vi "Load_Destinations.vi"(8 "error in (no error)":errorcluster, 11 "AB_Application in":refnum<class "AB_Application.lvclass">) -> (0 "error out":errorcluster, 3 "AB_Application out":refnum<class "AB_Application.lvclass">)   [LabVIEW 2020, in "AB_Application.lvclass"]
uses:
  <vilib>/AppBuilder/AB_Classes/Application/AB_Application.lvclass
  e:/builds/penguin/labview/branches/2020/dev/dist/vi.lib/AppBuilder/AB_Classes/TargetFile/AB_Targetfile.lvclass
  e:/builds/penguin/labview/branches/2020/dev/dist/vi.lib/AppBuilder/AB_Classes/Build/AB_Build.lvclass
  <vilib>/AppBuilder/AB_Classes/TargetFile/AB_Targetfile.lvclass
  <vilib>/AppBuilder/AB_Classes/Build/AB_Build.lvclass
  <vilib>/AppBuilder/AB_Classes/Destination/AB_Destination.lvclass
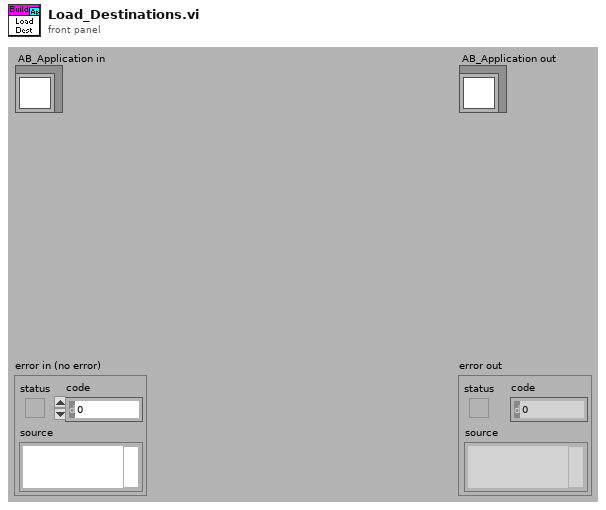
[diagram p1: front panel]
types:
  T1 = typedef "AB_Targetfile.ctl" = cluster{"targetfileName":string, "targetfileGUID":string, "enableDebugging":bool, "versionInfo":cluster{"productName":string, "legalCopyright":string, "companyName":string, "internalName":string, "fileDescription":string}, "eng_consolidatedTypeInfo":string, "fastFileFormat":bool, "eng_LEIFBuildData":u32, "versionIndependent":bool}
  T2 = typedef "AB_Build.ctl" = cluster{"buildSpecName":string, "buildSpecDescription":string, "destinations":refnum<class "AB_Destination.lvclass">[], "exclusionOption":T3, "defaultLanguage":string, "supportedLanguages":string[], "excludedDirectories":path[], "buildContext":refnum<vi>, "buildObject":T4, "preview":bool, "programatic":bool, "progressBarEvents":T5, "userLog_Path":path, "preActionID":string, "preAction_Path":path, "postActionID":string, "postAction_Path":path, "eng_checkForBrokenVIs?":bool, "eng_verboseLinkerErrors?":bool, "localDest_Path":path, "targetDest_Path":path, "removeVIObject":u16, "cache":refnum<class "PreviewCache.lvclass">, "use cache":bool, "previewCache_ID":string, "buildCache_ID":string, "eng_TempLocalDest_Path":path, "eng_collectDependencies?":bool, "versionInfo":cluster{"buildVersion":cluster{"major":u16, "minor":u16, "patch":u16, "build":u16}, "autoIncrement":bool}, "eng_enableVIChecksums":bool}
  T3 = typedef "AB_Exclusion_Option.ctl" = cluster{"typedefs":bool, "polymorphicVIs":bool, "unusedLibraryItems":bool, "modifyLibraryFile":bool, "edit-timeDependencies":bool, "inlineVIs":bool, "dependent PPLs":bool, "dependent DLLs":bool}
  T4 = typedef "ItemRef.ctl" = u64
  T5 = typedef "provcom_ProgressBar_Events.ctl" = cluster{"newJob":refnum<user-event>, "newItem":refnum<user-event>, "errorMsg":T6, "cancel":refnum<user-event>}
  T6 = typedef "mxLvBuildError.ctl" = refnum<user-event>
  T7 = typedef "AB_Destination.ctl" = cluster{"destName":string, "path":path, "libraryName":string, "preserveHierarchy":bool, "eng_inBuild":bool, "eng_libraryReference":refnum<vi>, "eng_restictAddToNewLibrary":bool}
  T8 = enum32{"invalid OS target", "Mac OS", "Windows 3.1", "Windows 95/NT", "Solaris 1", "Solaris 2", "HP-UX", "PowerMAX", "Linux", "Irix", "Rhapsody", "BeOS", "AIX", "OSF1", "VxWorks", "PharLap", "Carbon", "RTX", "Windows x64", "Linux x64", "Mac OS X x64"}
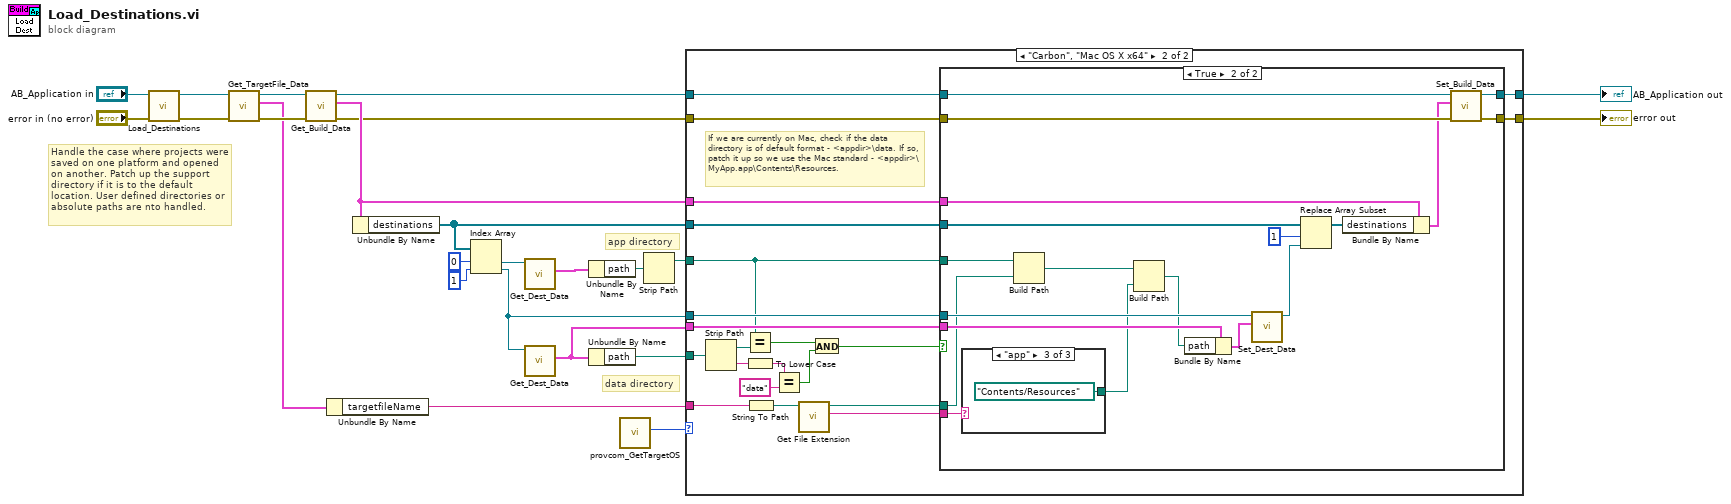
[diagram p0: block diagram]
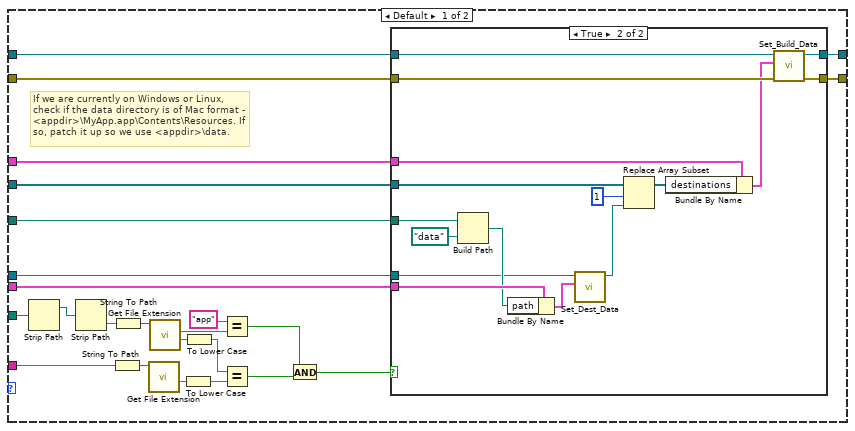
[diagram p2: hidden frame]
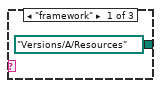
[diagram p5: hidden frame]
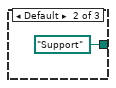
[diagram p6: hidden frame]
diagram:
  # "Handle the case where projects were saved on one platform and opened on another. Patch up the support directory if it is to the default location. User defined directories or absolute paths are nto handled."
  # "data directory"
  # "app directory"
  n1 = call-parent "Load_Destinations.vi"("error in (no error)"="error in (no error)", "AB_Build in"="AB_Application in") -> ("error out"=w3:errorcluster, "AB_Build out"=w5:refnum<class "AB_Application.lvclass">)  [unwired: 8 in]
  n2 = call <vilib>:"Get_TargetFile_Data.vi"("error in (no error)"=w3, "AB_Targetfile in"=w5) -> ("error out"=w2:errorcluster, "data"=w1:T1, "AB_Targetfile out"=w4:refnum<class "AB_Application.lvclass">)  [unwired: 7 in]
  n3 = call <vilib>:"Get_Build_Data.vi"("error in (no error)"=w2, "Class in"=w4) -> ("error out"=w10:errorcluster, "data"=w12:T2, "Class out"=w11:refnum<class "AB_Application.lvclass">)  [unwired: 7 in]
  n4 = Unbundle By Name(w1) -> ("targetfileName"=w13:string)
  n5 = Unbundle By Name(w12) -> ("destinations"=w16:refnum<class "AB_Destination.lvclass">[])
  n6 = Index Array(array=w16, index #1=0 ("index"), index #2=1 ("index")) -> (element #1=w20:refnum<class "AB_Destination.lvclass">, element #2=w6:refnum<class "AB_Destination.lvclass">)
  n7 = call <vilib>:"Get_Dest_Data.vi"("Class in"=w20) -> ("destName"=w21:T7)  [unwired: 8 in, 2 out]
  n8 = call <vilib>:"Get_Dest_Data.vi"("Class in"=w6) -> ("destName"=w7:T7)  [unwired: 8 in, 2 out]
  n9 = Unbundle By Name(w21) -> ("path"=w18:path)
  n10 = Unbundle By Name(w7) -> ("path"=w14:path)
  n11 = call <resource>:"provcom_GetTargetOS.vi"() -> ("App.TargetOS"=w17:T8)  [unwired: 11 in]
  n12 = Strip Path(path=w18) -> (stripped path=w15:path)  [unwired: 1 out]
  n13 = case shown="\"Carbon\", \"Mac OS X x64\"" w17 {
    tunnel: w16 -> [w32 w81]
    tunnel: w15 -> [w33 w77]
    tunnel: w14 -> [w48 w87]
    tunnel: w13 -> [w46 w70]
    tunnel: w12 -> [w38 w86]
    tunnel: w11 -> [w37 w85]
    tunnel: w10 -> [w36 w84]
    tunnel: [w35 w83] -> w9
    tunnel: [w34 w82] -> w8
    tunnel: w7 -> [w31 w80]
    tunnel: w6 -> [w30 w79]
    frame Default {
      # "If we are currently on Windows or Linux, check if the data directory is of Mac format - <appdir>\\MyApp.app\\Contents\\Resources. If so, patch it up so we use <appdir>\\data."
      n14 = Strip Path(path=w48) -> (stripped path=w47:path)  [unwired: 1 out]
      n15 = Strip Path(path=w47) -> (name=w40:string)  [unwired: 1 out]
      n16 = String To Path(string=w46) -> (path=w45:path)
      n17 = String To Path(string=w40) -> (path=w41:path)
      n18 = call <vilib>:"Get File Extension.vi"("file"=w45) -> ("filename without extension"=w44:string)  [unwired: 6 in, 4 out]
      n19 = call <vilib>:"Get File Extension.vi"("file"=w41) -> ("filename without extension"=w42:string, "lowercase file extension"=w29:string)  [unwired: 6 in, 3 out]
      n20 = To Lower Case(string=w44) -> (all lower case string=w43:string)
      n21 = To Lower Case(string=w42) -> (all lower case string=w39:string)
      n22 = Equal?(x="app", y=w29) -> (x = y?=w27:bool)
      n23 = Equal?(x=w39, y=w43) -> (x = y?=w26:bool)
      n24 = And(x=w27, y=w26) -> (x .and. y?=w25:bool)
      n25 = case shown="True" w25 {
        tunnel: w38 -> [_ w53]
        tunnel: w37 -> [w50 w66]
        tunnel: w36 -> [w49 w64]
        tunnel: [w50 w65] -> w35
        tunnel: [w49 w63] -> w34
        tunnel: w33 -> [_ w62]
        tunnel: w32 -> [_ w56]
        tunnel: w31 -> [_ w60]
        tunnel: w30 -> [_ w58]
        frame False {
        }
        frame True {
          n26 = Build Path(base path=w62, name or relative path=path "data" ("stripped path")) -> (appended path=w59:path)
          n27 = Bundle By Name(cluster=w60, "path"=w59) -> (w57:T7)
          n28 = call <vilib>:"Set_Dest_Data.vi"("destName"=w57, "Class in"=w58) -> ("Class out"=w55:refnum<class "AB_Destination.lvclass">)  [unwired: 8 in, 1 out]
          n29 = Replace Array Subset(array=w56, new element=w55, index=1) -> (w52:refnum<class "AB_Destination.lvclass">[])
          n30 = Bundle By Name(cluster=w53, "destinations"=w52) -> (w51:T2)
          n31 = call <vilib>:"Set_Build_Data.vi"("error in (no error)"=w64, "data"=w51, "Class in"=w66) -> ("error out"=w63:errorcluster, "Class out"=w65:refnum<class "AB_Application.lvclass">)  [unwired: 7 in]
        }
      }
    }
    frame "Carbon", "Mac OS X x64" {
      # "If we are currently on Mac, check if the data directory is of default format - <appdir>\\data. If so, patch it up so we use the Mac standard - <appdir>\\MyApp.app\\Contents\\Resources."
      n32 = Strip Path(path=w87) -> (stripped path=w78:path, name=w76:string)
      n33 = Equal?(x=w77, y=w78) -> (x = y?=w73:bool)
      n34 = To Lower Case(string=w76) -> (all lower case string=w75:string)
      n35 = String To Path(string=w70) -> (path=w69:path)
      n36 = Equal?(x=w75, y="data") -> (x = y?=w72:bool)
      n37 = call <vilib>:"Get File Extension.vi"("file"=w69) -> ("lowercase file extension"=w67:string, "dup file"=w68:path)  [unwired: 6 in, 3 out]
      n38 = And(x=w73, y=w72) -> (x .and. y?=w71:bool)
      n39 = case shown="True" w71 {
        tunnel: w86 -> [_ w97]
        tunnel: w85 -> [w89 w108]
        tunnel: w84 -> [w88 w106]
        tunnel: [w89 w107] -> w83
        tunnel: [w88 w105] -> w82
        tunnel: w77 -> [_ w104]
        tunnel: w81 -> [_ w100]
        tunnel: w80 -> [_ w103]
        tunnel: w79 -> [_ w102]
        tunnel: w68 -> [_ w92]
        tunnel: w67 -> [_ w91]
        frame False {
        }
        frame True {
          n40 = case shown="\"app\"" w91 {
            tunnel: [path "Versions/A/Resources" ("f") path "Support" ("f") path "Contents/Resources"] -> w90
            frame "framework" {
            }
            frame Default {
            }
            frame "app" {
            }
          }
          n41 = Build Path(base path=w104, name or relative path=w92) -> (appended path=w94:path)
          n42 = Build Path(base path=w94, name or relative path=w90) -> (appended path=w93:path)
          n43 = Bundle By Name(cluster=w103, "path"=w93) -> (w101:T7)
          n44 = call <vilib>:"Set_Dest_Data.vi"("destName"=w101, "Class in"=w102) -> ("Class out"=w99:refnum<class "AB_Destination.lvclass">)  [unwired: 8 in, 1 out]
          n45 = Replace Array Subset(array=w100, new element=w99, index=1) -> (w96:refnum<class "AB_Destination.lvclass">[])
          n46 = Bundle By Name(cluster=w97, "destinations"=w96) -> (w95:T2)
          n47 = call <vilib>:"Set_Build_Data.vi"("error in (no error)"=w106, "data"=w95, "Class in"=w108) -> ("error out"=w105:errorcluster, "Class out"=w107:refnum<class "AB_Application.lvclass">)  [unwired: 7 in]
        }
      }
    }
  }
  "error out" <- w8
  "AB_Application out" <- w9
